vi "Move_test_3Wheel.vi"() -> ()   [LabVIEW 2013]
panel:
  out "Voltage":dbl(graph)
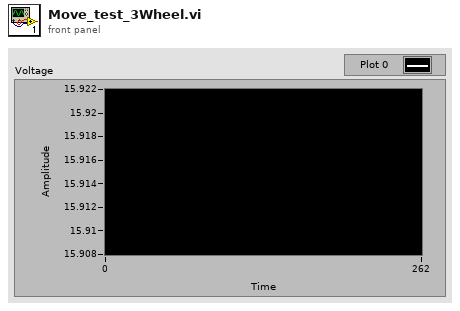
[diagram p1: front panel]
types:
  T1 = typedef "KNR3 Reference.ctl" = cluster{"FPGA Session":refnum<class "FPGA Interface Base.lvclass">, "Resource":T2}
  T2 = typedef "Resource.ctl" = enum16{"KNRm_DDRC", "KNRm_DDDD", "KNRm_DDDR", "KNRm_DDDC", "KNR"}
  T3 = cluster{"Mode":enum16{"FRWD", "TURFIX", "TURNOF"}, "Dir":enum16{"Left", "Right"}, "Pcmd":dbl, "Vcmd":dbl}
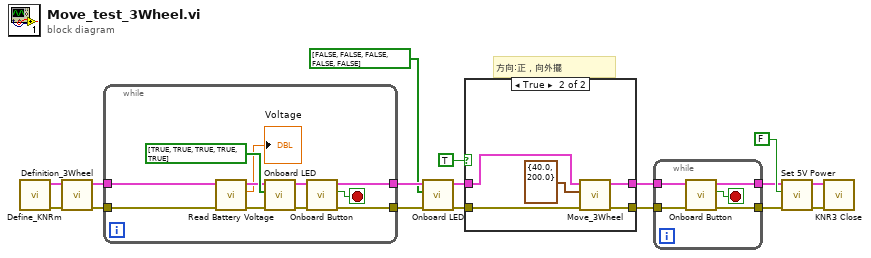
[diagram p0: block diagram]
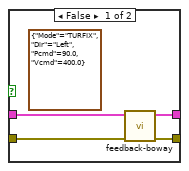
[diagram p2: hidden frame]
diagram:
  # "方向:正，向外擺"
  n1 = call "Define_KNRm.vi"() -> ("error out"=w5:errorcluster, "KNR out"=w6:T1)  [unwired: 10 in]
  n2 = call "Definition_3Wheel.vi"("error in (no error)"=w5, "KNR in"=w6) -> ("error out"=w7:errorcluster, "KNR out"=w8:T1)  [unwired: 8 in]
  n3 = while {
    tunnel: [w27] -> w17
    tunnel: [w25] -> w15
    tunnel: w8 -> [w19]
    tunnel: w7 -> [w18]
    stop <- w28 stop-if-true
    n4 = call <userlib>:"Read Battery Voltage.vi"("error in (no error)"=w18, "KNR in"=w19) -> ("error out"=w21:errorcluster, "Voltage"=→"Voltage":dbl, "KNR out"=w22:T1)  [unwired: 7 in]
    n5 = call <userlib>:"Onboard LED.vi"("error in (no error)"=w21, "LED List"=bool[] [TRUE, TRUE, TRUE, TRUE, TRUE], "KNR in"=w22) -> ("error out"=w26:errorcluster, "KNR out"=w24:T1)  [unwired: 7 in]
    n6 = call <userlib>:"Onboard Button.vi"("error in (no error)"=w26, "KNR in"=w24) -> ("error out"=w25:errorcluster, "value"=w28:bool, "KNR out"=w27:T1)  [unwired: 7 in]
  }
  n7 = call <userlib>:"Onboard LED.vi"("error in (no error)"=w15, "LED List"=bool[] [FALSE, FALSE, FALSE, FALSE, FALSE], "KNR in"=w17) -> ("error out"=w9:errorcluster, "KNR out"=w10:T1)  [unwired: 7 in]
  n8 = case shown="True" TRUE {
    tunnel: w9 -> [w32 w36]
    tunnel: [w31 w34] -> w3
    tunnel: w10 -> [w30 w37]
    tunnel: [w29 w35] -> w4
    frame False {
      (unwired) T3 {"Mode"=enum."TURFIX", "Dir"=enum."Left", "Pcmd"=90.0, "Vcmd"=400.0} ("Move")
      n9 = call "feedback-boway.vi"("error in (no error)"=w32, "KNR in"=w30) -> ("error out"=w31:errorcluster, "KNR out"=w29:T1)  [unwired: 7 in, 1 out]
    }
    frame True {
      n10 = call "Move_3Wheel.vi"("error in (no error)"=w36, "Cluster"=cluster{"UDmm)":dbl, "Vcmd":dbl} {"UDmm)"=40.0, "Vcmd"=200.0}, "KNR in"=w37) -> ("error out"=w34:errorcluster, "KNR out"=w35:T1)  [unwired: 7 in]
    }
  }
  n11 = while {
    tunnel: w4 -> [w42]
    tunnel: w3 -> [w41]
    tunnel: [w40] -> w2
    tunnel: [w39] -> w1
    stop <- w38 stop-if-true
    n12 = call <userlib>:"Onboard Button.vi"("error in (no error)"=w41, "KNR in"=w42) -> ("error out"=w39:errorcluster, "value"=w38:bool, "KNR out"=w40:T1)  [unwired: 7 in]
  }
  n13 = call <userlib>:"Set 5V Power.vi"("error in (no error)"=w1, "5V Power(T)"=FALSE, "KNR in"=w2) -> ("error out"=w14:errorcluster, "KNR out"=w13:T1)  [unwired: 7 in]
  n14 = call <userlib>:"KNR3 Close.vi"("error in (no error)"=w14, "KNR in"=w13) -> ()  [unwired: 9 in, 1 out]
